vi "close.vi"(8 "error in (no error)":errorcluster, 11 "SoundAO in":refnum<class "SoundAO.lvclass">) -> (0 "error out":errorcluster)   [LabVIEW 2011, in "Hardware.lvlib" / "Channels.lvlib" / "SoundAO.lvclass"]
uses:
  SoundAO.lvclass
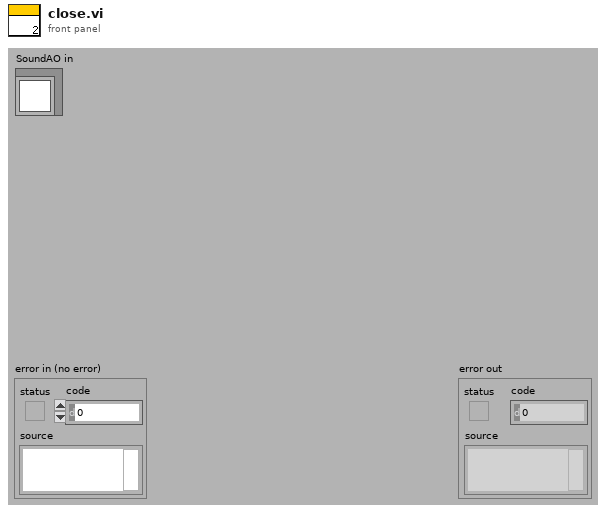
[diagram p1: front panel]
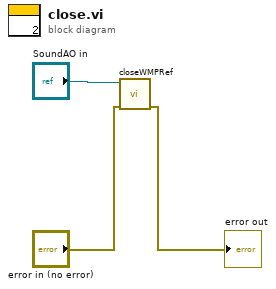
[diagram p0: block diagram]
diagram:
  n1 = call "closeWMPRef.vi"("error in (no error)"="error in (no error)", "SoundAO in"="SoundAO in") -> ("error out"=→"error out":errorcluster)  [unwired: 8 in, 1 out]
